vi "accumulator system.vi"(3 "Sequence x[n]":dbl[](array[numeric])=[1.0, 2.0, 3.0, 4.0, 5.0, 6.0, 7.0]) -> (0 "Waveform of Accumulated sequence A[n]":dbl[](graph)=[1.0, 3.0, 6.0, 10.0, 15.0, 21.0, 28.0], 1 "Accumulated sequence A[n] = Sum(k: k ( -infinity to n) x[k]":dbl[](array[numeric])=[1.0, 3.0, 6.0, 10.0, 15.0, 21.0, 28.0], 2 "Waveform of sequence x[n]":dbl[](graph)=[1.0, 2.0, 3.0, 4.0, 5.0, 6.0, 7.0])   [LabVIEW 2009]
panel:
  # "Assignment 5: Exercise 4-1: Accmulator System"
  # "A5_Ex_4_1_accumulator system.vi"
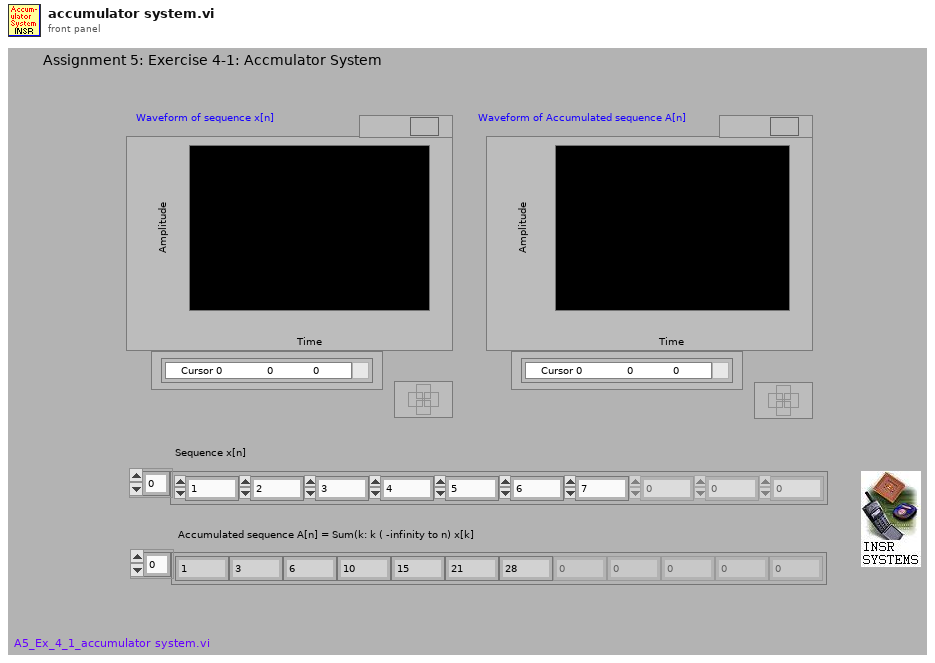
[diagram p1: front panel]
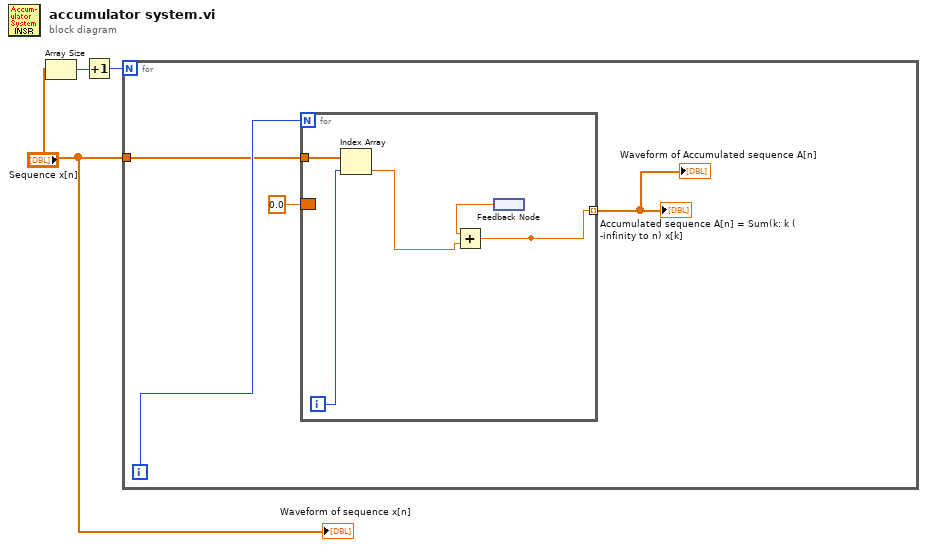
[diagram p0: block diagram]
diagram:
  n1 = Array Size(array="Sequence x[n]") -> (size(s)=w3:i32)
  n2 = Increment(x=w3) -> (x+1=w2:i32)
  n3 = for {
    N: w2 -> [_]
    tunnel: "Sequence x[n]" -> [w6]
    i -> [w7]
    n4 = for {
      N: w7 -> [_]
      tunnel: w6 -> [w12]
      tunnel: [w8] -> w4 mode=indexing
      border: 0.0 -> [_]
      i -> [w10]
      n5 = Index Array "Index Array"(array=w12, index=w10) -> (element=w11:dbl)
      n6 = feedback #1() -> (w9:dbl)
      n7 = Add(x=w9, y=w11) -> (x+y=w8:dbl)
    }
    "Accumulated sequence A[n] = Sum(k: k ( -infinity to n) x[k]" <- w4
    "Waveform of Accumulated sequence A[n]" <- w4
  }
  "Waveform of sequence x[n]" <- "Sequence x[n]"
